vi "RP set frequency batch.vi"(8 "Error In":errorcluster, 10 "Frequency":dbl[](array[numeric]), 11 "connection ID":refnum<k5>) -> (0 "Error Out":errorcluster, 2 "Phase words sent":u32[](array[numeric]), 3 "connection ID out":refnum<k5>)   [LabVIEW 2015]
uses:
  RP Command.ctl
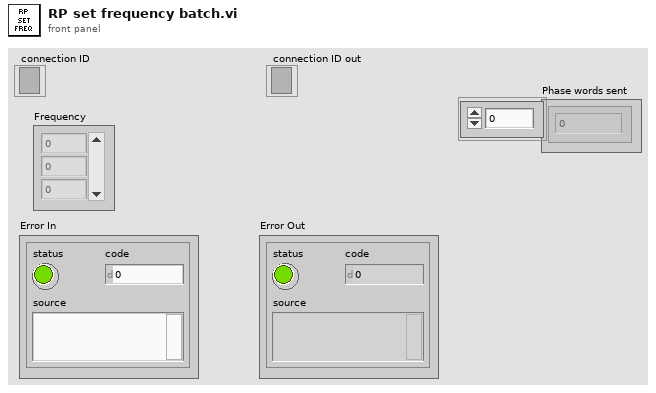
[diagram p1: front panel]
types:
  T1 = enum16{"big-endian, network order", "native, host order", "little-endian"}
  T2 = typedef "RP Command.ctl" = enum16{"Set frequency", "Arm and get data", "Stop server", "Get status", "Get temperature", "Set decimation", "Arm", "Software trigger", "Get whole buffer", "Get chunk", "System call", "Get config", "Set config", "Read FIFO", "Play pattern", "Set frequency batch"}
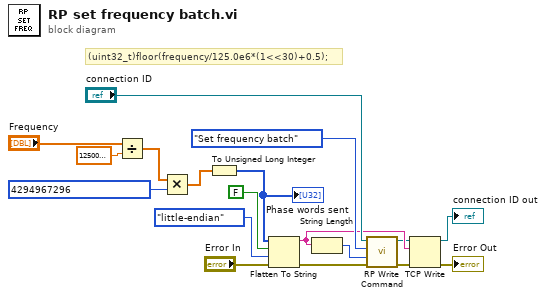
[diagram p0: block diagram]
diagram:
  # "(uint32_t)floor(frequency/125.0e6*(1<<30)+0.5);"
  n1 = Divide(x="Frequency", y=125000000.0) -> (x/y=w16:dbl[])
  n2 = Multiply(x=w16, y=i64 4294967296) -> (x*y=w15:dbl[])
  n3 = To Unsigned Long Integer(number=w15) -> (unsigned 32bit integer=w10:u32[])
  "Phase words sent" <- w10
  n4 = Flatten To String(anything=w10, prepend array or string size? (T)=FALSE, byte order (0:big-endian, network order)=T1."little-endian", error in (no error)="Error In") -> (data string=w8:string, error out=w3:errorcluster)  [unwired: 1 out]
  n5 = String Length(string=w8) -> (length=w1:i32)
  n6 = call "RP Write Command.vi"("Error In"=w3, "Command payload"=w1, "Command number"=RP_Command."Set frequency batch", "connection ID"="connection ID") -> ("Error Out"=w2:errorcluster, "connection ID out"=w7:refnum<k5>)  [unwired: 5 in, 1 out]
  n7 = TCP Write(connection ID=w7, data in=w8, error in (no error)=w2) -> (connection ID out=→"connection ID out":refnum<k5>, error out=→"Error Out":errorcluster)  [unwired: 1 in, 1 out]
